vi "Register Temporary Feeds.vi"(8 "error in (no error)":errorcluster, 10 "Feeds":T2[](array[typedef]), 11 "Feed Manager State Data in":T1) -> (0 "error out":errorcluster, 3 "Feed Manager State Data out":T1)   [LabVIEW 2014]
doc: "Temporarily register any feeds that are not already registered."
uses:
  Feed Info.ctl
  Feed Manager State Data.ctl
  UI references.ctl
  <vilib>/National Instruments/NIPM API (Beta)/NIPM_API.lvlib
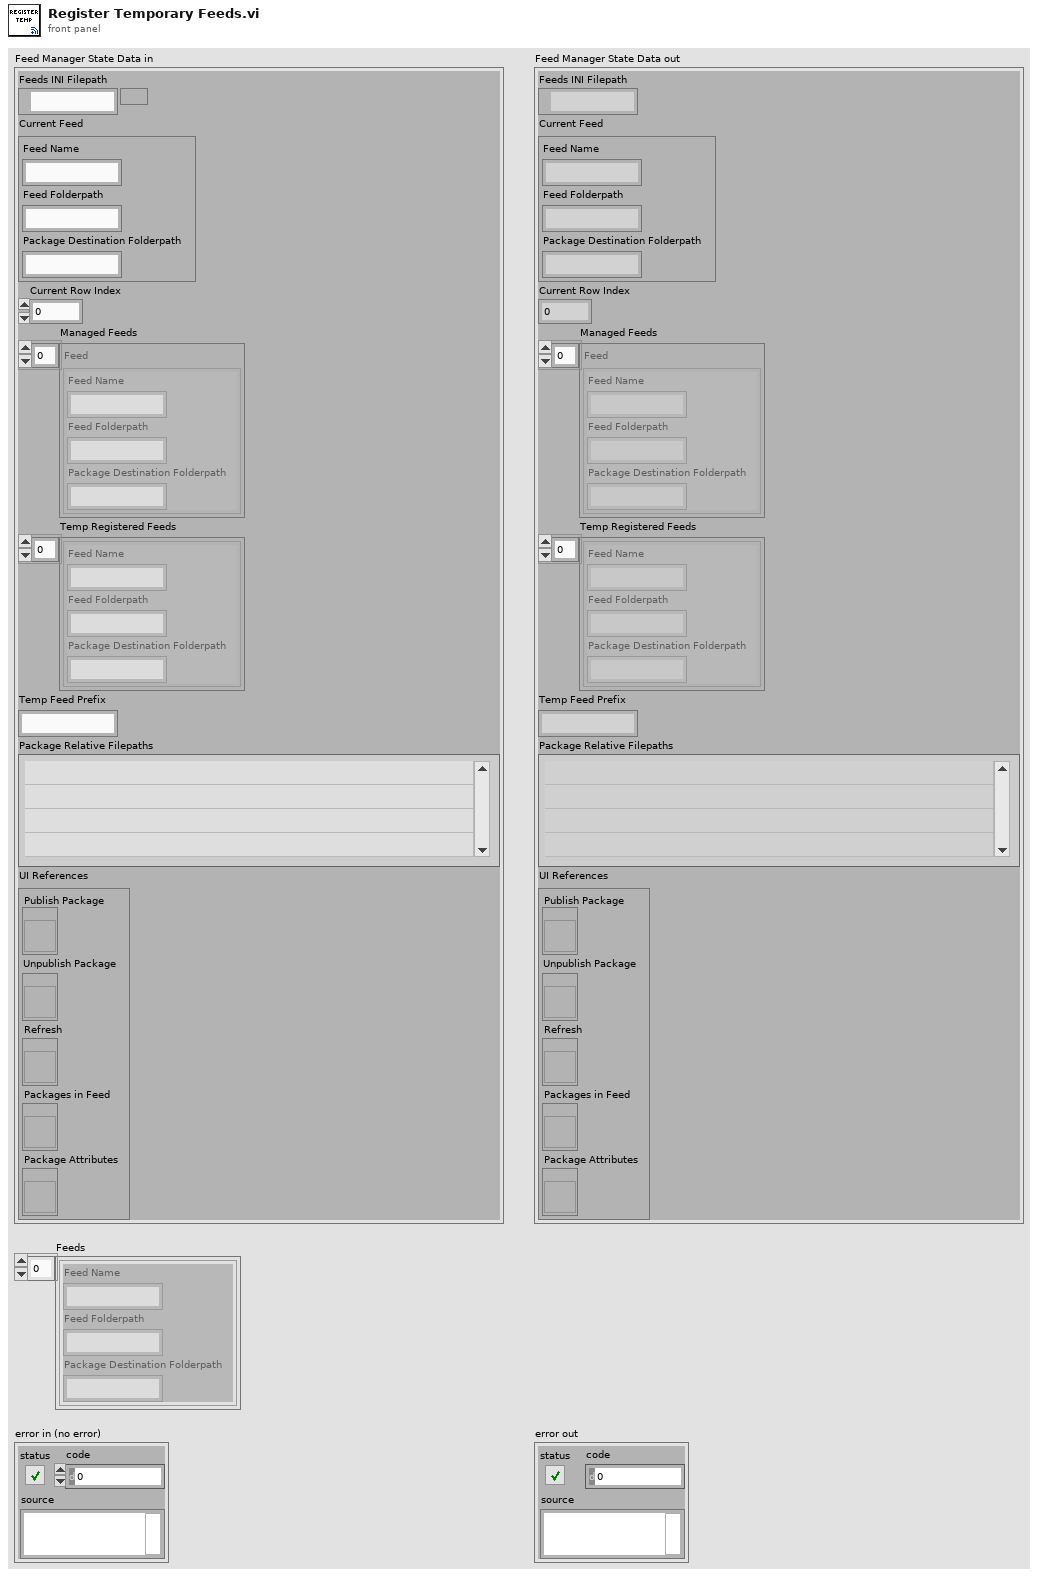
[diagram p1: front panel]
types:
  T1 = typedef "Feed Manager State Data.ctl" = cluster{"Feeds INI Filepath":path, "Current Feed":T2, "Current Row Index":i32, "Managed Feeds":T2[], "Temp Registered Feeds":T2[], "Temp Feed Prefix":string, "Package Relative Filepaths":path[], "UI References":T3}
  T2 = typedef "Feed Info.ctl" = cluster{"Feed Name":string, "Feed Folderpath":string, "Package Destination Folderpath":string}
  T3 = typedef "UI references.ctl" = cluster{"Publish Package":refnum<vi>, "Unpublish Package":refnum<vi>, "Refresh":refnum<vi>, "Packages in Feed":refnum<vi>, "Package Attributes":refnum<vi>}
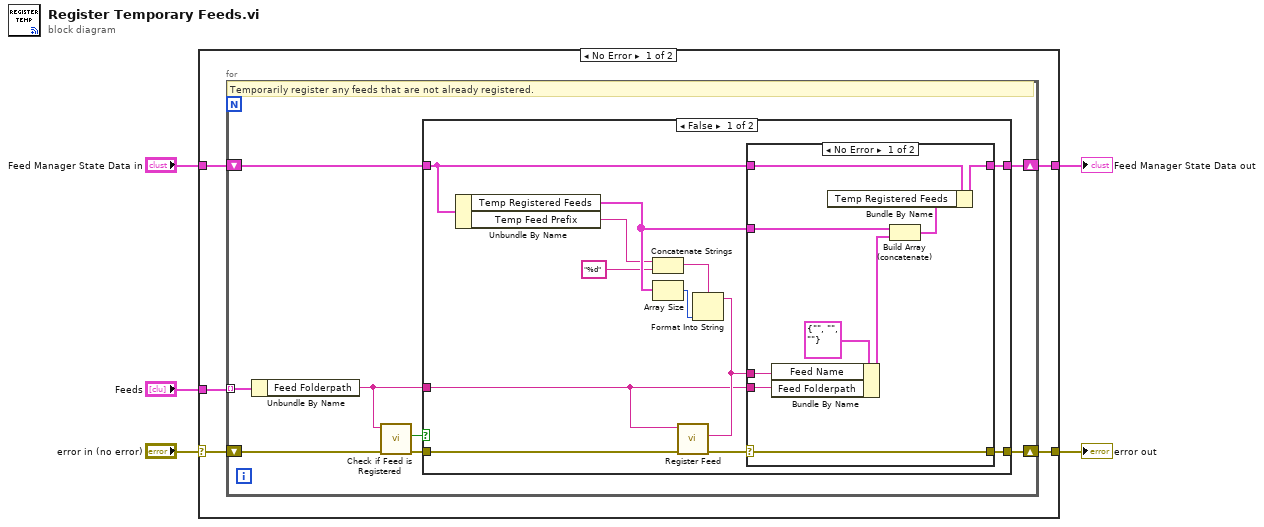
[diagram p0: block diagram]
diagram:
  n1 = case shown="No Error" "error in (no error)" {
    selector: "error in (no error)" -> [w6 w45]
    tunnel: "Feeds" -> [w10 _]
    tunnel: "Feed Manager State Data in" -> [w9 w44]
    tunnel: [w8 w44] -> w3
    tunnel: [w7 w45] -> w2
    frame No Error {
      n2 = for {
        shift-right: [w16] -> w7
        shift-left: w6 -> [w18]
        tunnel: w10 -> [w17] mode=indexing
        shift-right: [w14] -> w8
        shift-left: w9 -> [w15]
        # "Temporarily register any feeds that are not already registered."
        n3 = Unbundle By Name(w17) -> ("Feed Folderpath"=w11:string)
        n4 = call <vilib>:"Check if Feed is Registered.vi"("error in"=w18, "feed URI"=w11) -> ("error out"=w13:errorcluster, "feed URI registered?"=w12:bool)  [unwired: 6 in, 2 out]
        n5 = case shown="False" w12 {
          tunnel: w13 -> [w29 w42]
          tunnel: [w25 w42] -> w16
          tunnel: w15 -> [w28 w43]
          tunnel: [w27 w43] -> w14
          tunnel: w11 -> [w22 _]
          frame False {
            n6 = Unbundle By Name(w28) -> ("Temp Registered Feeds"=w24:T2[], "Temp Feed Prefix"=w21:string)
            n7 = Concatenate Strings(w21, "%d" ("string")) -> (w19:string)
            n8 = Array Size(array=w24) -> (size(s)=w30:i32)
            n9 = Format Into String(format string=w19, w30) -> (resulting string=w23:string)  [unwired: 2 in, 1 out]
            n10 = call <vilib>:"Register Feed.vi"("error in"=w29, "feed name"=w23, "feed URI"=w22) -> ("error out"=w26:errorcluster)  [unwired: 7 in, 1 out]
            n11 = case shown="No Error" w26 {
              selector: w26 -> [w37 w40]
              tunnel: w28 -> [w39 w41]
              tunnel: [w38 w41] -> w27
              tunnel: [w37 w40] -> w25
              tunnel: w24 -> [w36 _]
              tunnel: w23 -> [w33 _]
              tunnel: w22 -> [w32 _]
              frame No Error {
                n12 = Bundle By Name(cluster=T2 {"Feed Name"="", "Feed Folderpath"="", "Package Destination Folderpath"=""} ("Temp Registered Feeds"), "Feed Name"=w33, "Feed Folderpath"=w32) -> (w31:T2)
                n13 = Build Array (concatenate)(w36, w31) -> (w35:T2[])
                n14 = Bundle By Name(cluster=w39, "Temp Registered Feeds"=w35) -> (w38:T1)
              }
              frame Error {
              }
            }
          }
          frame True {
          }
        }
      }
    }
    frame Error {
    }
  }
  "Feed Manager State Data out" <- w3
  "error out" <- w2
